vi "wdt_analog.vi"() -> ()   [LabVIEW 2019]
uses:
  <vilib>/Analysis/NI_AALBase.lvlib
panel:
  out "Error Out":errorcluster
  in  "TDMS File":path=path "C:/Python/projects/nitdms/tests/tdms_files/wdt_analog.tdms"
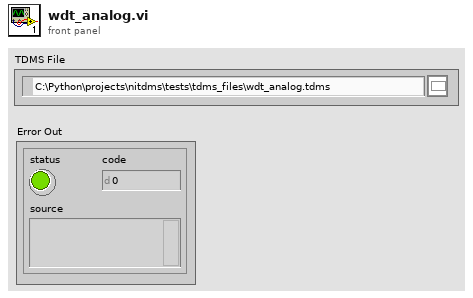
[diagram p1: front panel]
types:
  T1 = enum16{"open", "open or create", "create or replace", "create", "open (read-only)"}
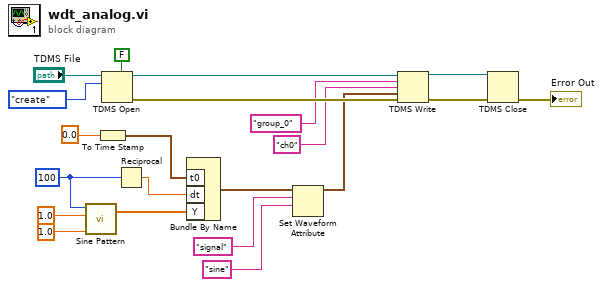
[diagram p0: block diagram]
diagram:
  w15 = 100 ("samples")
  n1 = call <vilib>:"Sine Pattern.vi"("cycles"=1.0, "amplitude"=1.0, "samples"=w15) -> ("Sinusoidal Pattern"=w16:dbl[])  [unwired: 1 in, 1 out]
  n2 = To Time Stamp(1:0.0) -> (0:w2:timestamp)
  n3 = TDMS Open(5:FALSE ("create index file? (T)"), 10:T1."create" ("operation (0:open)"), 11:"TDMS File") -> (0:w11:errorcluster, 3:w10:refnum<k34>)  [unwired: 4 in]
  n4 = Reciprocal(x=w15) -> (1/x=w14:dbl)
  n5 = Bundle By Name("t0"=w2, "dt"=w14, "Y"=w16) -> (w13:waveform(dbl))  [unwired: 1 in]
  n6 = Set Waveform Attribute(5:"sine" ("name"), 6:"signal" ("name"), 7:w13) -> (3:w8:waveform(dbl))  [unwired: 1 in, 2 out]
  n7 = TDMS Write(0:w10, 5:"group_0" ("name"), 7:"ch0" ("name"), 9:w8, 11:w11) -> (4:w6:refnum<k34>, 15:w7:errorcluster)  [unwired: 1 in, 2 out]
  n8 = TDMS Close(8:w7, 11:w6) -> (0:→"Error Out":errorcluster)  [unwired: 1 out]
